vi "Exercise 5.1 - Creating Shared Variables.vi"() -> ()   [LabVIEW 2012]
panel:
  in  "stop":bool
  out "Boolean 3":bool
  out "Boolean 2":bool
  in  "Boolean":bool
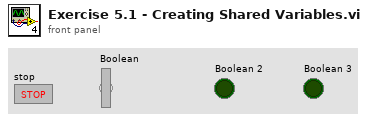
[diagram p1: front panel]
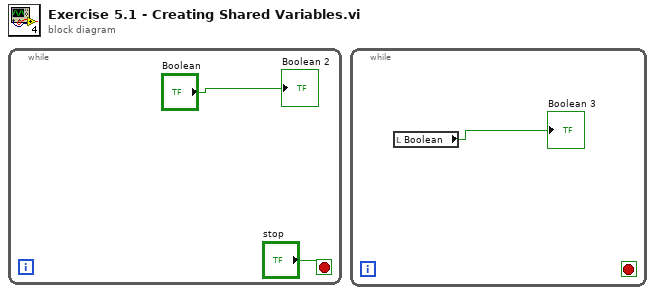
[diagram p0: block diagram]
diagram:
  n1 = while {
    stop <- "stop" stop-if-true
    "Boolean 2" <- "Boolean"
  }
  n2 = while {
    stop <- _ stop-if-true
    n3 = local read "Boolean"() -> (→"Boolean 3":bool)
  }
